vi "Counts Per Second to RPM.vi"(10 "Counts/Rev":dbl, 11 "Counts/Second":dbl) -> (3 "RPM":dbl)   [LabVIEW 2013]
doc: "Takes in Counts/Second and divides it by Counts/Revs. Returns the RPM"
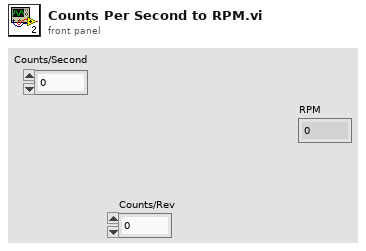
[diagram p1: front panel]
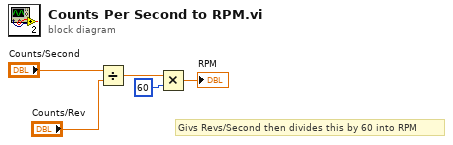
[diagram p0: block diagram]
diagram:
  # "Givs Revs/Second then divides this by 60 into RPM"
  n1 = Divide(x="Counts/Second", y="Counts/Rev") -> (x/y=w3:dbl)
  n2 = Multiply(x=w3, y=60) -> (x*y=→"RPM":dbl)
